vi "String to 2D Array.vi"(8 "error in (no error)":errorcluster, 10 "String":string) -> (0 "error out":errorcluster, 2 "2D Array":string[][](array[string]))   [LabVIEW 2016, in "Webscraper.lvlib"]
uses:
  Webscraper.lvlib
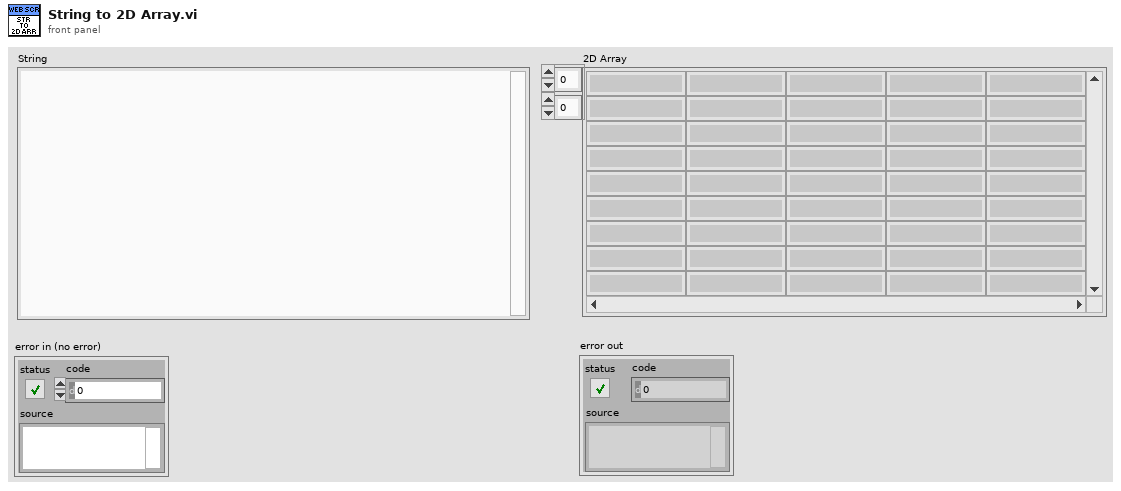
[diagram p1: front panel]
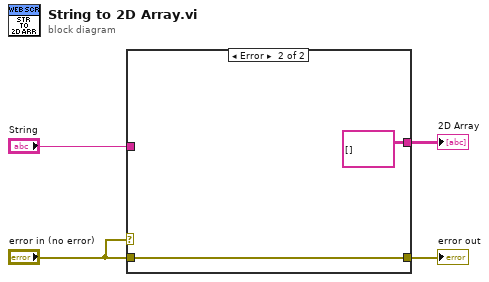
[diagram p0: block diagram]
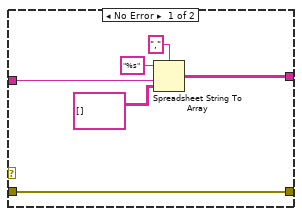
[diagram p2: hidden frame]
diagram:
  n1 = case shown="Error" "error in (no error)" {
    tunnel: [w10 string[][] []] -> w4
    tunnel: "error in (no error)" -> [w6 w11]
    tunnel: [w6 w11] -> w3
    tunnel: "String" -> [w5 _]
    frame No Error {
      n2 = Spreadsheet String To Array(delimiter (Tab)=",", format string="%s", spreadsheet string=w5, array type (2D Dbl)=string[][] []) -> (array=w10:string[][])
    }
    frame Error {
    }
  }
  "2D Array" <- w4
  "error out" <- w3
